vi "My Check Fit Convergence.vi"(0 "Chi 2":dbl, 1 "Lambda":dbl=-1.0, 5 "Parameters":dbl[](array[numeric]), 7 "gradient":dbl[](array[numeric]), 9 "my stopping criteria":T1={"function tolerance"=1e-06, "parameter tolerance"=1e-06, "max iterations"=0, "max function calls"=0, "gradient tolerance"=0.0, "max time (sec)"=1000.0, "initial tick count"=0, "min lambda"=1e-06, "max lambda"=1e-06}, 11 "Error In":errorcluster, 12 "current iteration":i32, 13 "number of function evaluations":i32) -> (3 "|Delta Chi 2|/Chi 2":dbl, 4 "stop?":bool, 6 "|Delta Chi 2|":dbl, 10 "Max |Delta a| /|a|":dbl, 15 "error out":errorcluster)   [LabVIEW 2019]
uses:
  My Fit Stopping Criteria.ctl
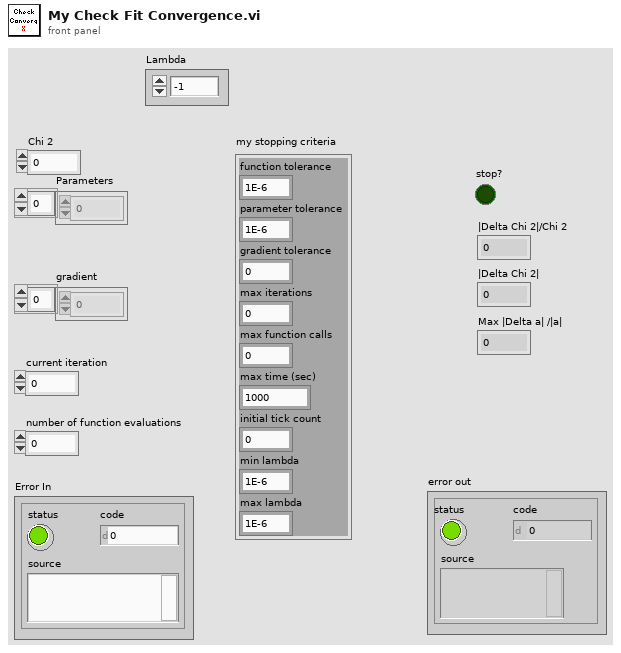
[diagram p1: front panel]
types:
  T1 = typedef "My Fit Stopping Criteria.ctl" = cluster{"function tolerance":dbl, "parameter tolerance":dbl, "max iterations":i32, "max function calls":i32, "gradient tolerance":dbl, "max time (sec)":dbl, "initial tick count":u32, "min lambda":dbl, "max lambda":dbl}
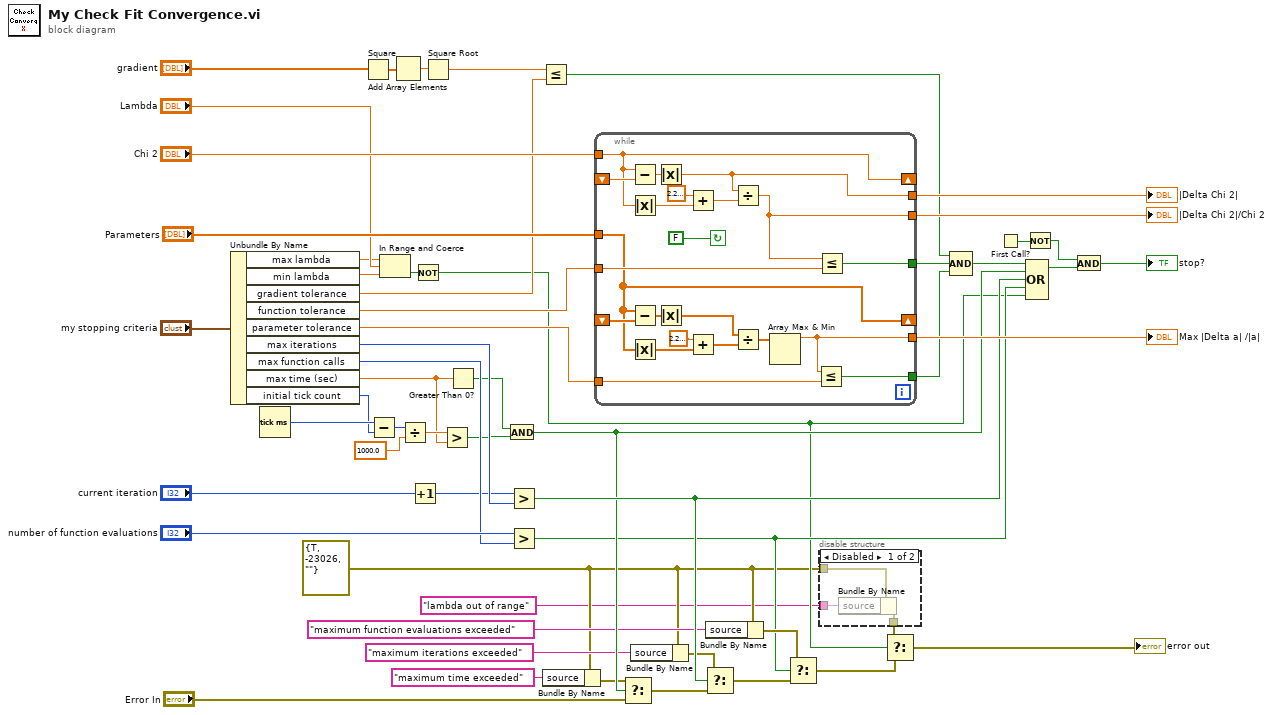
[diagram p0: block diagram]
diagram:
  w2 = errorcluster {"status"=TRUE, "code"=-23026, "source"=""} ("error out")
  n1 = Unbundle By Name("my stopping criteria") -> ("max lambda"=w15:dbl, "min lambda"=w14:dbl, "gradient tolerance"=w29:dbl, "function tolerance"=w41:dbl, "parameter tolerance"=w40:dbl, "max iterations"=w39:i32, "max function calls"=w38:i32, "max time (sec)"=w17:dbl, "initial tick count"=w21:u32)
  n2 = Tick Count (ms)() -> (millisecond timer value=w22:u32)
  n3 = Square(x="gradient") -> (x^2=w32:dbl[])
  n4 = Subtract(x=w22, y=w21) -> (x-y=w20:u32)
  n5 = In Range and Coerce(upper limit=w15, x="Lambda", lower limit=w14) -> (In Range?=w13:bool)  [unwired: 1 out]
  n6 = Add Array Elements(numeric array=w32) -> (sum=w31:dbl)
  n7 = Divide(x=w20, y=1000.0) -> (x/y=w18:dbl)
  n8 = Increment(x="current iteration") -> (x+1=w35:i32)
  n9 = Not(x=w13) -> (.not. x?=w4:bool)
  n10 = Square Root(x=w31) -> (sqrt(x)=w30:dbl)
  n11 = Greater?(x=w18, y=w17) -> (0:w16:bool)
  n12 = Greater Than 0?(x=w17) -> (x > 0?=w24:bool)
  n13 = And(x=w24, y=w16) -> (x .and. y?=w23:bool)
  n14 = Greater?(x=w35, y=w39) -> (0:w25:bool)
  n15 = Greater?(x="number of function evaluations", y=w38) -> (0:w5:bool)
  n16 = Less Or Equal?(x=w30, y=w29) -> (x <= y?=w28:bool)
  n17 = Bundle By Name(cluster=w2, "source"="maximum time exceeded") -> (w11:errorcluster)
  n18 = while {
    shift-right: [w74] -> _
    shift-left: _ -> [w75]
    tunnel: "Chi 2" -> [w74]
    tunnel: [w58] -> w43
    tunnel: "Parameters" -> [w57]
    shift-right: [w57] -> _
    shift-left: _ -> [w77]
    tunnel: [w59] -> w42
    tunnel: w41 -> [w64]
    tunnel: w40 -> [w63]
    tunnel: [w66] -> w50
    tunnel: [w76] -> w49
    tunnel: [w60] -> w48
    stop <- FALSE continue-if-true
    n19 = Subtract(x=w74, y=w75) -> (x-y=w67:dbl)
    n20 = Absolute Value(x=w74) -> (abs(x)=w73:dbl)
    n21 = Subtract(x=w57, y=w77) -> (x-y=w68:dbl[])
    n22 = Absolute Value(x=w57) -> (abs(x)=w71:dbl[])
    n23 = Absolute Value(x=w67) -> (abs(x)=w66:dbl)
    n24 = Absolute Value(x=w68) -> (abs(x)=w65:dbl[])
    n25 = Add(x=2.220446049250313e-16 ("machine eps"), y=w73) -> (x+y=w72:dbl)
    n26 = Add(x=2.220446049250313e-16 ("machine eps"), y=w71) -> (x+y=w70:dbl[])
    n27 = Divide(x=w66, y=w72) -> (x/y=w60:dbl)
    n28 = Divide(x=w65, y=w70) -> (x/y=w69:dbl[])
    n29 = Array Max & Min(array=w69) -> (max value=w76:dbl)  [unwired: 3 out]
    n30 = Less Or Equal?(x=w76, y=w63) -> (x <= y?=w59:bool)
    n31 = Less Or Equal?(x=w60, y=w64) -> (x <= y?=w58:bool)
  }
  "|Delta Chi 2|" <- w50
  "Max |Delta a| /|a|" <- w49
  "|Delta Chi 2|/Chi 2" <- w48
  n32 = Select(t=w11, s=w23, f="Error In") -> (s? t:f=w27:errorcluster)
  n33 = Bundle By Name(cluster=w2, "source"="maximum iterations exceeded") -> (w8:errorcluster)
  n34 = Select(t=w8, s=w25, f=w27) -> (s? t:f=w26:errorcluster)
  n35 = Bundle By Name(cluster=w2, "source"="maximum function evaluations exceeded") -> (w6:errorcluster)
  n36 = Select(t=w6, s=w5, f=w26) -> (s? t:f=w12:errorcluster)
  n37 = disable-structure shown="Disabled" {
    disable-tunnel: [w81 _] -> w3
    disable-tunnel: w2 -> [w80 _]
    disable-tunnel: "lambda out of range" ("source") -> [w79 _]
    frame Disabled {
      n38 = Bundle By Name(cluster=w80, "source"=w79) -> (w81:errorcluster)
    }
    frame Enabled {
    }
  }
  n39 = Select(t=w3, s=w4, f=w12) -> (s? t:f=→"error out":errorcluster)
  n40 = Compound Arithmetic op=AND(w28, w43, w42) -> (w33:bool)
  n41 = First Call?() -> (First Call?: T/F=w37:bool)
  n42 = Not(x=w37) -> (.not. x?=w36:bool)
  n43 = Compound Arithmetic op=OR(w33, w23, w25, w5, w4) -> (w34:bool)
  n44 = And(x=w36, y=w34) -> (x .and. y?=→"stop?":bool)
